vi "Generate Serial String.vi"(0 "Motor ID":u8, 5 "Command":u8, 7 "Address":u8, 9 "Parameters":string, 11 "Error in (no error)":errorcluster) -> (4 "Command to Serial":string, 15 "error out":errorcluster)   [LabVIEW 2016, in "Dynamixel Motor.lvlib"]
doc: "Generates a valid serial string that can be sent to the motor(s). This is a Low-Level VI that is used by other VIs."
uses:
  Dynamixel Motor.lvlib
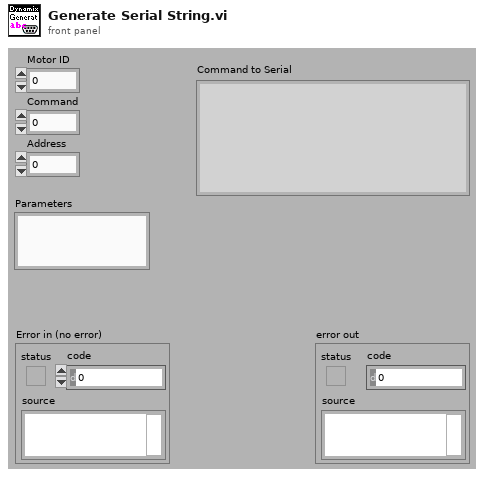
[diagram p1: front panel]
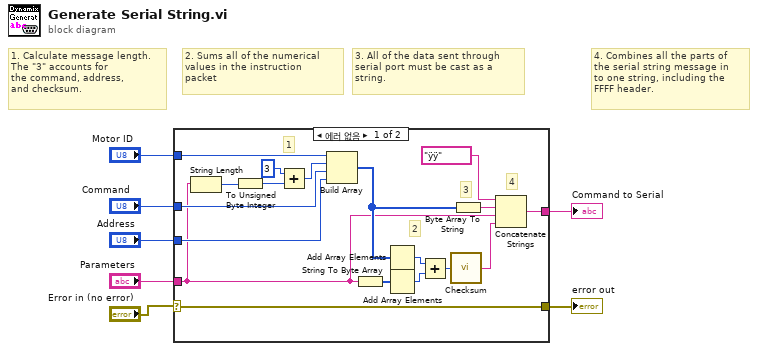
[diagram p0: block diagram]
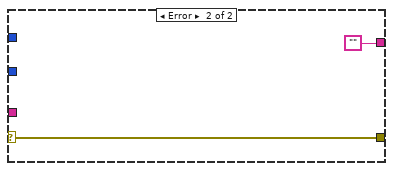
[diagram p2: hidden frame]
diagram:
  # "2. Sums all of the numerical \nvalues in the instruction \npacket"
  # "1. Calculate message length.\nThe \"3\" accounts for\nthe command, address,\nand checksum."
  # "3. All of the data sent through \nserial port must be cast as a \nstring."
  # "4. Combines all the parts of \nthe serial string message in \nto one string, including the \nFFFF header."
  n1 = case shown="에러 없음" "Error in (no error)" {
    selector: "Error in (no error)" -> [w13 w27]
    tunnel: "Address" -> [w18 _]
    tunnel: "Command" -> [w19 _]
    tunnel: "Motor ID" -> [w21 _]
    tunnel: [w22 ""] -> w4
    tunnel: [w13 w27] -> w3
    tunnel: "Parameters" -> [w12 _]
    frame No Error {
      # "4"
      # "3"
      # "2"
      # "1"
      n2 = String Length(string=w12) -> (length=w9:i32)
      n3 = To Unsigned Byte Integer(number=w9) -> (unsigned 8bit integer=w8:u8)
      n4 = Add(x=u8 3, y=w8) -> (x+y=w20:u8)
      n5 = Build Array(w21, w20, w19, w18) -> (w14:u8[])
      n6 = String To Byte Array(string=w12) -> (unsigned byte array=w11:u8[])
      n7 = Add Array Elements(numeric array=w14) -> (sum=w17:u8)
      n8 = Add Array Elements(numeric array=w11) -> (sum=w10:u8)
      n9 = Add(x=w17, y=w10) -> (x+y=w16:u8)
      n10 = call "Checksum.vi"("Sum of bytes"=w16) -> ("Checksum String"=w23:string)
      n11 = Byte Array To String(unsigned byte array=w14) -> (string=w15:string)
      n12 = Concatenate Strings("ÿÿ", w15, w12, w23) -> (w22:string)
    }
    frame Error {
    }
  }
  "Command to Serial" <- w4
  "error out" <- w3
